vi "Quick Usb Read Data.vi"(8 "error in (no error)":errorcluster, 9 "length":u32, 10 "data":string, 11 "hDevice":u32) -> (0 "error out":errorcluster, 1 "length out":u32, 2 "data out":string, 3 "hDevice out":u32, 5 "function return":i32)   [LabVIEW 2011, in "QuickUSB.lvlib"]
doc: "QUSBLIB QRETURN QuickUsbReadData(\n QHANDLE hDevice, \n PQBYTE data, \n PQULONG length\n);"
uses:
  QuickUSB.lvlib
  QuickUSB.dll
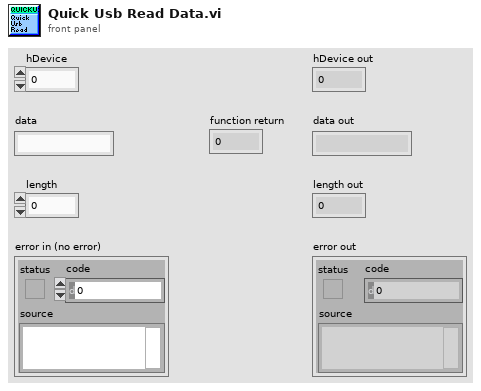
[diagram p1: front panel]
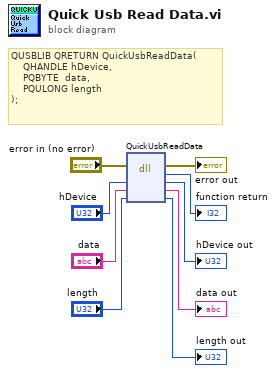
[diagram p0: block diagram]
diagram:
  # "QUSBLIB QRETURN QuickUsbReadData(\n    QHANDLE hDevice, \n    PQBYTE  data, \n    PQULONG length\n);"
  n1 = dll-call lib="C:/QuickUSB/QuickUSB.*" fn="QuickUsbReadData"(error in="error in (no error)", "hDevice"="hDevice", "data"="data", "length"="length") -> (error out=→"error out":errorcluster, →"function return":i32, "hDevice"=→"hDevice out":u32, "data"=→"data out":string, "length"=→"length out":u32)  [unwired: 2 in, 1 out]
